vi "Serialize.vi"(8 "error in":errorcluster, 9 "OwningElement in":refnum<k20>, 10 "Document in":refnum<k20>, 11 "MeasureLimit in":refnum<class "MeasureLimit.lvclass">) -> (0 "error out":errorcluster, 1 "OwningElement out":refnum<k20>, 2 "Document out":refnum<k20>, 3 "MeasureLimit out":refnum<class "MeasureLimit.lvclass">)   [LabVIEW 2021, in "ProligentXMLGenerator.lvlib" / "MeasureLimit.lvclass"]
uses:
  MeasureLimit.lvclass
  MeasureLimit.lvclass/MeasureLimit.ctl
  <vilib>/xml/NI_XML.lvlib
  Base/DOMSupport/DOMSupport.lvlib
  Model/CustomData/CustomData.lvclass
  <vilib>/xml/Close Reference(Node).vi
  Base/Attribute/Attribute.lvclass
  Base/NonEmptyString_2000/NonEmptyString_2000.lvclass
  C:/Projects/proligent-xml-generator-labview/src/ProligentXMLGenerator/Base/NonEmptyString/NonEmptyString.lvclass
  C:/Projects/proligent-xml-generator-labview/src/ProligentXMLGenerator/Base/String/String.lvclass
  C:/Projects/proligent-xml-generator-labview/src/ProligentXMLGenerator/Base/Attribute/Attribute.lvclass
  C:/Projects/proligent-xml-generator-labview/src/ProligentXMLGenerator/Base/NonEmptyString_2000/NonEmptyString_2000.lvclass
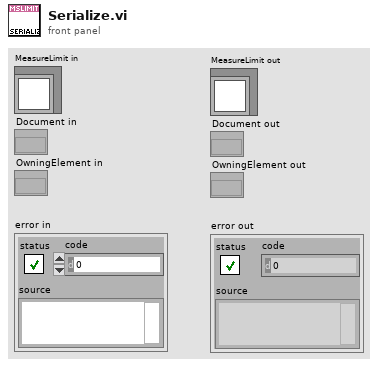
[diagram p1: front panel]
types:
  T1 = typedef "ProligentXMLGenerator.lvlib/MeasureLimit.lvclass/Data.ctl" = cluster{"Name":string, "CustomData":refnum<class "CustomData.lvclass">, "LimitExpression":refnum<class "NonEmptyString_2000.lvclass">}
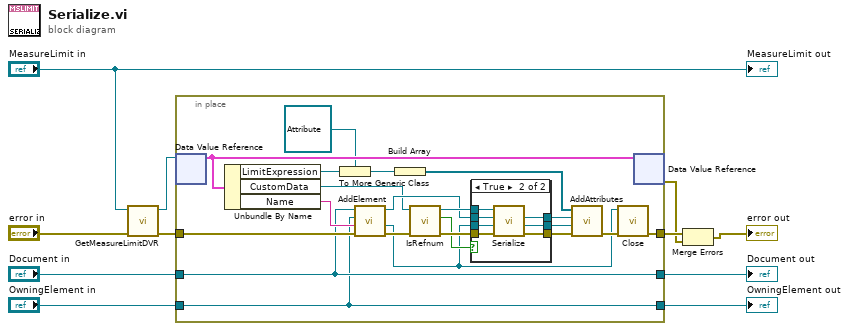
[diagram p0: block diagram]
diagram:
  n1 = call "GetMeasureLimitDVR.vi"("error in"="error in", "MeasureLimit"="MeasureLimit in") -> ("error out"=w4:errorcluster, "DVRReference"=w3:refnum<data-value>)  [unwired: 8 in]
  n2 = in-place "In Place Element Structure" {
    in-place-border: [w31] -> w5
    in-place-border: "Document in" -> [w18]
    in-place-border: w4 -> [w21]
    in-place-border: "OwningElement in" -> [w17]
    in-place-border: [w17] -> w7
    in-place-border: [w18] -> w6
    n3 = in-place-dvr #1(w3) -> (w32:T1)  [unwired: 1 out]
    n4 = Unbundle By Name(w32) -> ("LimitExpression"=w14:refnum<class "NonEmptyString_2000.lvclass">, "CustomData"=w20:refnum<class "CustomData.lvclass">, "Name"=w19:string)
    n5 = To More Generic Class(target class=refnum<class "Attribute.lvclass"> refnum ("ProligentResultProcessor:Attribute"), reference=w14) -> (generic class reference=w13:refnum<class "Attribute.lvclass">)
    n6 = call "AddElement.vi"("error in"=w21, "Name"=w19, "OwningElement in"=w17, "Document in"=w18) -> ("error out"=w22:errorcluster, "NewElement"=w15:refnum<k20>, "Document out"=w26:refnum<k20>)  [unwired: 4 in, 1 out]
    n7 = Build Array(w13) -> (w27:refnum<class "Attribute.lvclass">[])
    n8 = call "IsRefnum.vi"("error in"=w22, "CustomDataType in"=w20) -> ("error out"=w30:errorcluster, "IsRefnum"=w28:bool, "CustomDataType out"=w29:refnum<class "CustomData.lvclass">)  [unwired: 7 in]
    n9 = case shown="True" w28 {
      tunnel: w26 -> [w34 w42]
      tunnel: w30 -> [w35 w41]
      tunnel: w15 -> [w33 w40]
      tunnel: [w35 w39] -> w23
      tunnel: w29 -> [_ w38]
      tunnel: [w34 w37] -> w24
      tunnel: [w33 w36] -> w25
      frame False {
      }
      frame True {
        n10 = call "Serialize.vi"("error in"=w41, "OwningElement in"=w40, "Document in"=w42, "CustomDataType in"=w38) -> ("error out"=w39:errorcluster, "OwningElement out"=w36:refnum<k20>, "Document out"=w37:refnum<k20>)  [unwired: 4 in, 1 out]
      }
    }
    n11 = call "AddAttributes.vi"("error in"=w23, "OwningElement in"=w25, "Document in"=w24, "Attributes"=w27) -> ("error out"=w16:errorcluster)  [unwired: 5 in, 2 out]
    n12 = call-poly <vilib>:"Close.vi"("error in (no error)"=w16, "node"=w15) -> ("error out"=w31:errorcluster)  [unwired: 7 in]
    n13 = in-place-dvr #1(w32) -> (w2:errorcluster)  [unwired: 1 out]
  }
  "Document out" <- w6
  "OwningElement out" <- w7
  n14 = Merge Errors(w5, w2) -> (→"error out":errorcluster)
  "MeasureLimit out" <- "MeasureLimit in"
